vi "FTR Type DB Manager.vi"(5 "Command":T2, 6 "Local Data in":T3, 7 "UI Refs":T1, 8 "error in (no error)":errorcluster, 10 "Mouse Position (Start)":cluster{"X":i32, "Y":i32}) -> (0 "error out":errorcluster, 4 "Local Data out":T3)   [LabVIEW 2024]
uses:
  Controls/RVHR - Local Data.ctl
  Controls/Test Cluster.ctl
  Controls/Excluded Information.ctl
  Controls/Language.ctl
  Controls/Device_Type.ctl
  <vilib>/Utility/miscctls.llb/LVRectTypeDef.ctl
  <vilib>/Utility/miscctls.llb/LVBoundsTypeDef.ctl
  Controls/DB FTR Commands.ctl
  Controls/RVHR - UI Refs.ctl
  <vilib>/drjdpowell/SQLite Library/SQL Connection/Open (path).vi
  <vilib>/drjdpowell/SQLite Library/SQL Connection/Open (string).vi
  <vilib>/AdvancedString/Path To Command Line String.vi
  <vilib>/drjdpowell/SQLite Library/SQL Connection/Execute SQL.vi
  <vilib>/drjdpowell/SQLite Library/SQL Connection/Execute SQL (No results).vi
  <vilib>/drjdpowell/SQLite Library/SQL Connection/Execute SQL (Single Integer).vi
  <vilib>/drjdpowell/SQLite Library/SQL Connection/Connection.lvclass
  <vilib>/drjdpowell/SQLite Library/SQLite.lvlib
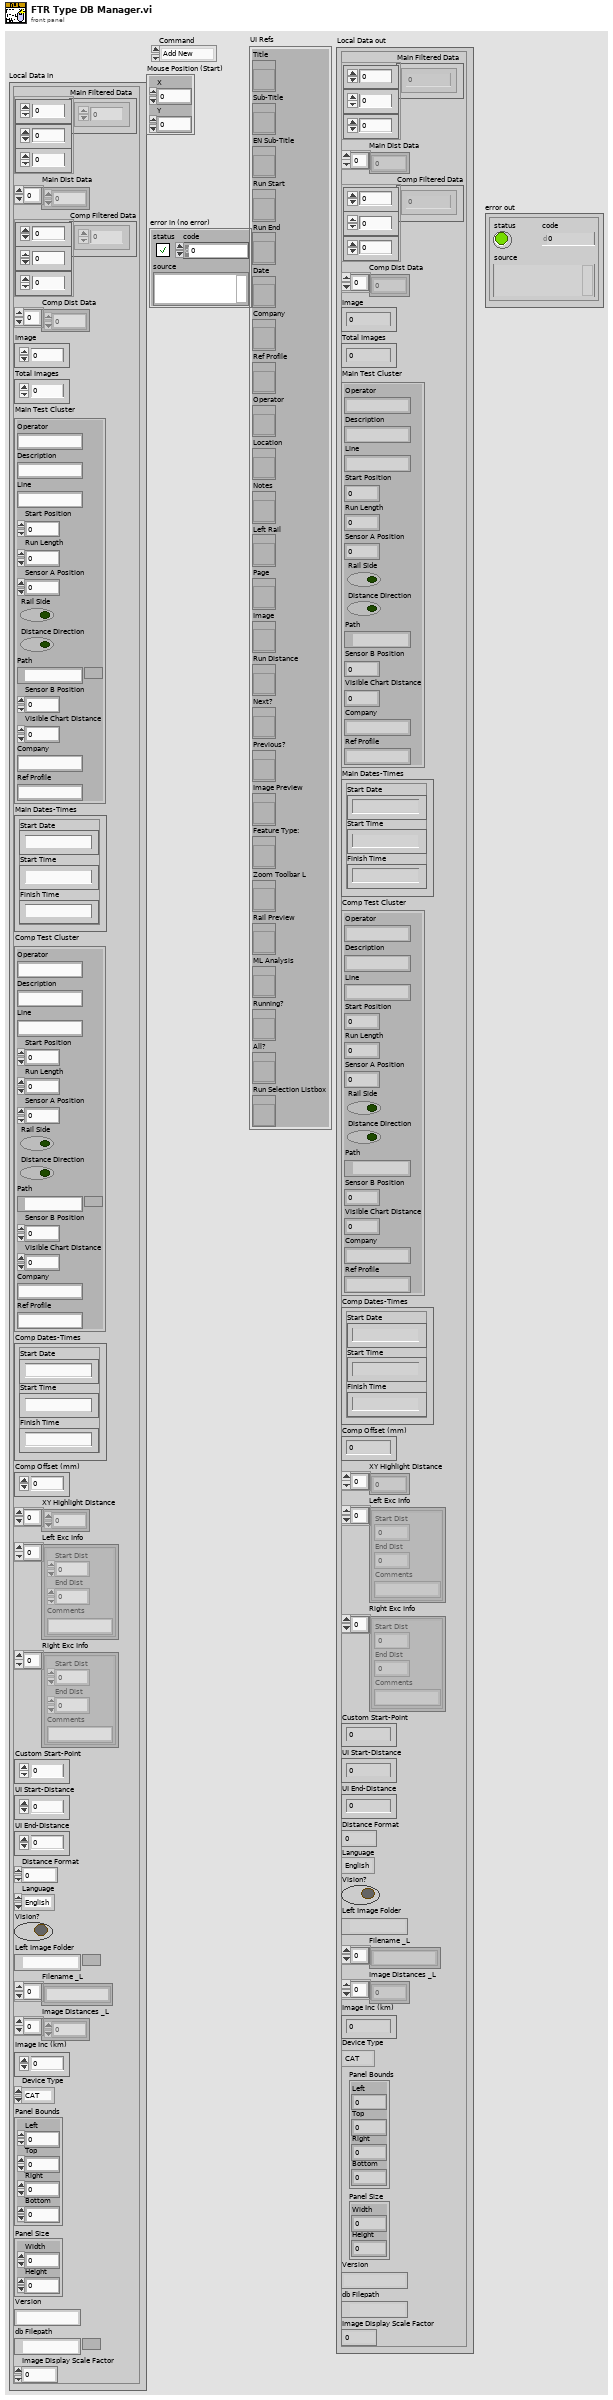
[diagram p1: front panel]
types:
  T1 = typedef "RVHR - UI Refs.ctl" = cluster{"Title":refnum<vi>, "Sub-Title":refnum<vi>, "EN Sub-Title":refnum<vi>, "Run Start":refnum<vi>, "Run End":refnum<vi>, "Date":refnum<vi>, "Company":refnum<vi>, "Ref Profile":refnum<vi>, "Operator":refnum<vi>, "Location":refnum<vi>, "Notes":refnum<vi>, "Left Rail":refnum<vi>, "Page":refnum<vi>, "Image":refnum<vi>, "Run Distance":refnum<vi>, "Next?":refnum<vi>, "Previous?":refnum<vi>, "Image Preview":refnum<vi>, "Feature Type:":refnum<vi>, "Zoom Toolbar L":refnum<vi>, "Rail Preview":refnum<vi>, "ML Analysis":refnum<vi>, "Running?":refnum<vi>, "All?":refnum<vi>, "Run Selection Listbox":refnum<vi>}
  T2 = typedef "DB FTR Commands.ctl" = enum16{"Add New", "Get", "Update"}
  T3 = typedef "RVHR - Local Data.ctl" = cluster{"Main Filtered Data":dbl[][][], "Main Dist Data":dbl[], "Comp Filtered Data":dbl[][][], "Comp Dist Data":dbl[], "Image":u16, "Total Images":u16, "Main Test Cluster":T4, "Main Dates-Times":cluster{"Start Date":string, "Start Time":string, "Finish Time":string}, "Comp Test Cluster":T4, "Comp Dates-Times":cluster{"Start Date":string, "Start Time":string, "Finish Time":string}, "Comp Offset (mm)":i64, "XY Highlight Distance":dbl[], "Left Exc Info":T5[], "Right Exc Info":T5[], "Custom Start-Point":dbl, "UI Start-Distance":dbl, "UI End-Distance":dbl, "Distance Format":u8, "Language":T6, "Vision?":bool, "Left Image Folder":path, "Filename _L":string[], "Image Distances _L":dbl[], "Image Inc (km)":dbl, "Device Type":T7, "Panel Bounds":T8, "Panel Size":T9, "Version":string, "db Filepath":path, "Image Display Scale Factor":dbl}
  T4 = typedef "Test Cluster.ctl" = cluster{"Operator":string, "Description":string, "Line":string, "Start Position":dbl, "Run Length":dbl, "Sensor A Position":dbl, "Rail Side":bool, "Distance Direction":bool, "Path":path, "Sensor B Position":dbl, "Visible Chart Distance":dbl, "Company":string, "Ref Profile":string}
  T5 = typedef "Excluded Information.ctl" = cluster{"Start Dist":dbl, "End Dist":dbl, "Comments":string}
  T6 = typedef "Language.ctl" = enum16{"English", "Chinese", "German"}
  T7 = typedef "Device_Type.ctl" = enum16{"CAT", "Bi-CAT", "YRCA", "RCA", "RV-HR", "TV-HR"}
  T8 = typedef "LVRectTypeDef.ctl" = cluster{"Left":i16, "Top":i16, "Right":i16, "Bottom":i16}
  T9 = typedef "LVBoundsTypeDef.ctl" = cluster{"Width":u32, "Height":u32}
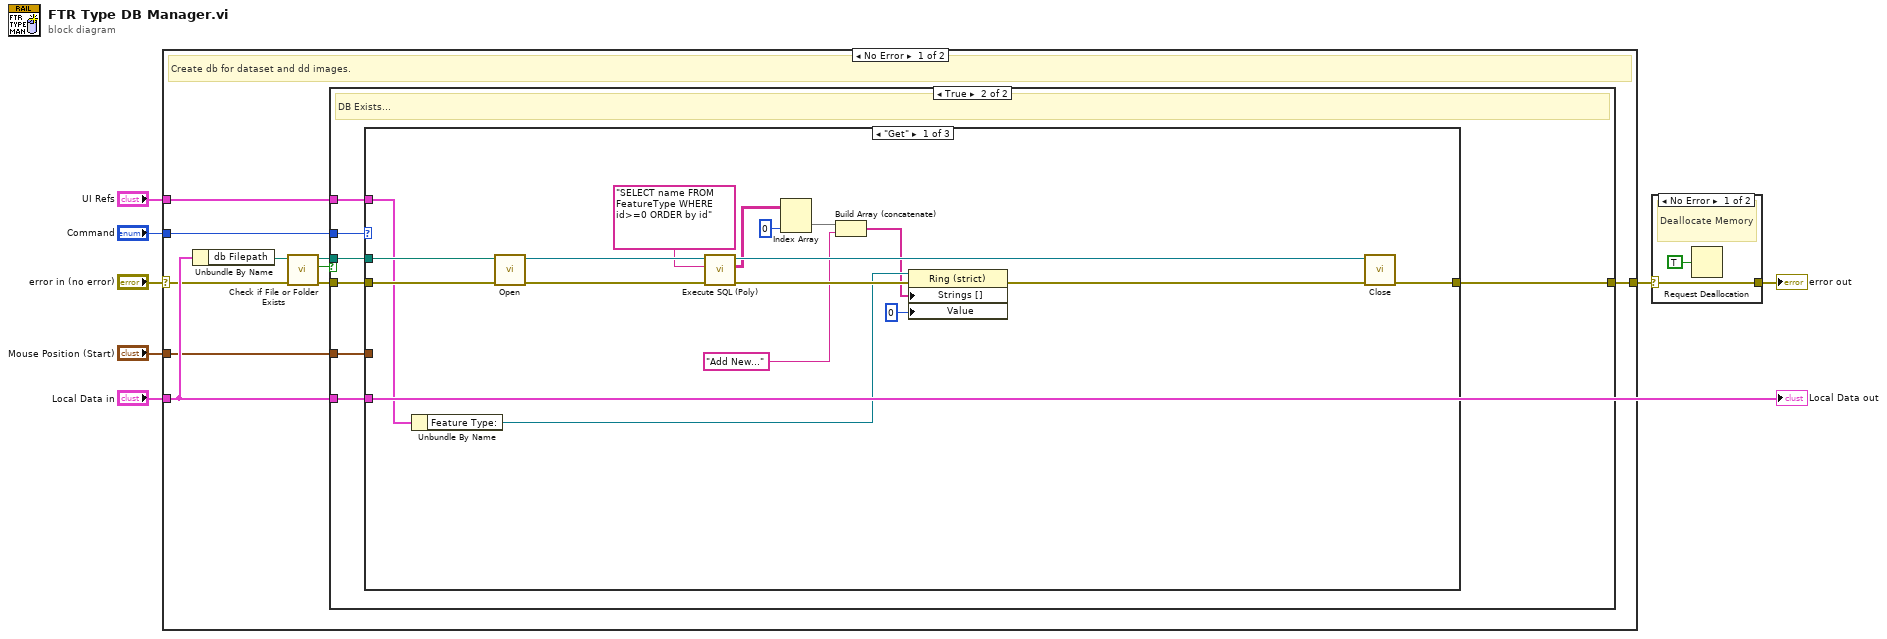
[diagram p0: block diagram]
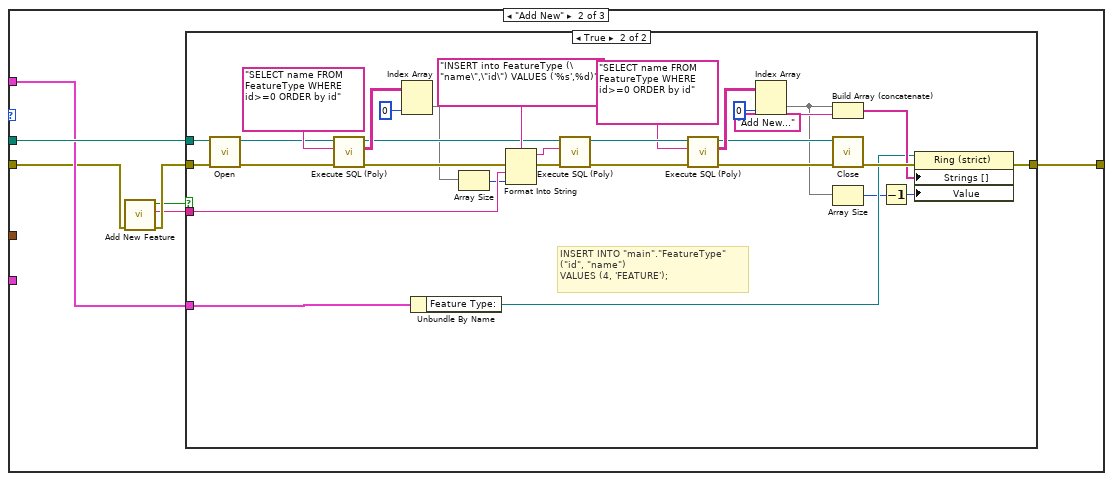
[diagram p4: hidden frame]
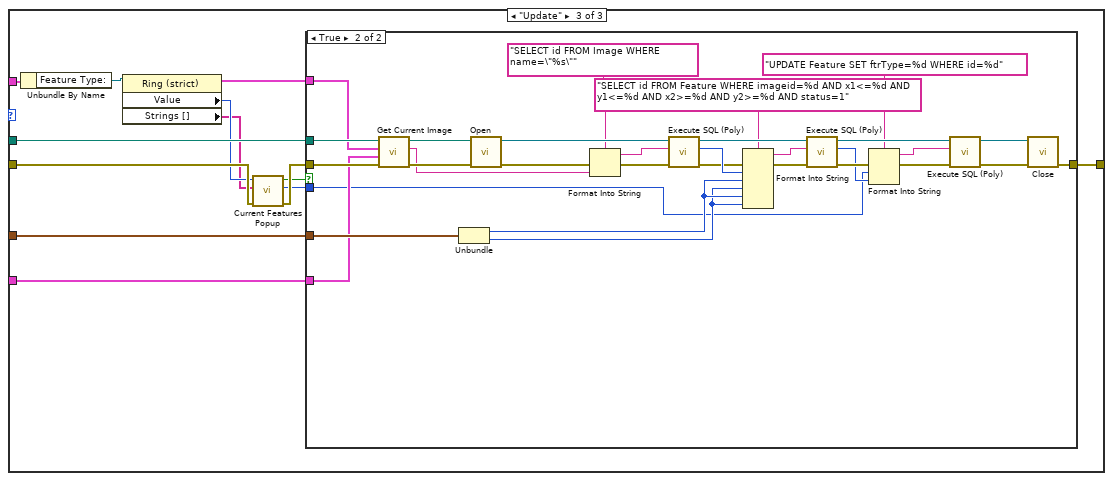
[diagram p6: hidden frame]
diagram:
  n1 = case shown="No Error" "error in (no error)" {
    selector: "error in (no error)" -> [w12 w124]
    tunnel: [w14 w124] -> w2
    tunnel: "Local Data in" -> [w13 _]
    tunnel: "Command" -> [w10 _]
    tunnel: "UI Refs" -> [w9 _]
    tunnel: "Mouse Position (Start)" -> [w8 _]
    frame No Error {
      # "Create db for dataset and dd images."
      n2 = Unbundle By Name(w13) -> ("db Filepath"=w11:path)
      n3 = call <vilib>:"Check if File or Folder Exists.vi"("error in (no error)"=w12, "path"=w11) -> ("error out"=w15:errorcluster, "file or folder exists?"=w17:bool, "dup path"=w16:path)  [unwired: 7 in]
      n4 = case shown="True" w17 {
        tunnel: w16 -> [_ w22]
        tunnel: w15 -> [w18 w23]
        tunnel: w13 -> [_ w25]
        tunnel: [w18 w24] -> w14
        tunnel: w10 -> [_ w21]
        tunnel: w9 -> [_ w20]
        tunnel: w8 -> [_ w19]
        frame False {
          # "Does not exist. Do nothing..."
        }
        frame True {
          # "DB Exists..."
          n5 = case shown="\"Get\"" w21 {
            tunnel: w25 -> [_ _ w81]
            tunnel: [w41 w49 w92] -> w24
            tunnel: w23 -> [w40 w46 w90]
            tunnel: w22 -> [w39 w48 w91]
            tunnel: w20 -> [w34 w47 w82]
            tunnel: w19 -> [_ _ w83]
            frame "Get" {
              n6 = Unbundle By Name(w34) -> ("Feature Type:"=w32:refnum<vi>)
              n7 = call-poly <vilib>:"Open.vi"("error in (no error)"=w40, "db file"=w39) -> ("error out"=w37:errorcluster, "SQLite Connection"=w42:refnum<class "Connection.lvclass">)  [unwired: 8 in]
              n8 = call-poly <vilib>:"Execute SQL (Poly).vi"("error in (no error)"=w37, "SQL"="SELECT name FROM FeatureType WHERE id>=0 ORDER by id" ("format string"), "SQLite Connection in"=w42) -> ("error out"=w35:errorcluster, "Result Set"=w30:string[][], "SQLite Connection"=w38:refnum<class "Connection.lvclass">)  [unwired: 5 in, 1 out]
              n9 = Index Array(array=w30, index (col)=0 ("disabled index (col)")) -> (element=w29:string[])  [unwired: 1 in]
              n10 = Build Array (concatenate)(w29, "Add New...") -> (w27:string[])
              n11 = property class="Ring (strict)"(reference=w32, error in=w35, "Strings []"=w27, "Value"=u16 0) -> (error out=w33:errorcluster)  [unwired: 1 out]
              n12 = call-dynamic "Close.vi"("error in (no error)"=w33, "SQLite Connection in"=w38) -> ("error out"=w41:errorcluster)  [unwired: 9 in]
            }
            frame "Add New" {
              n13 = call "Add New Feature.vi"("error in"=w46) -> ("error out"=w45:errorcluster, "New Feature"=w43:string, "Add New?"=w44:bool)  [unwired: 8 in]
              n14 = case shown="True" w44 {
                tunnel: [w50 w80] -> w49
                tunnel: w45 -> [w50 w79]
                tunnel: w48 -> [_ w78]
                tunnel: w47 -> [_ w69]
                tunnel: w43 -> [_ w67]
                frame False {
                }
                frame True {
                  # "INSERT INTO \"main\".\"FeatureType\"\n(\"id\", \"name\")\nVALUES (4, 'FEATURE');"
                  n15 = call-poly <vilib>:"Open.vi"("error in (no error)"=w79, "db file"=w78) -> ("error out"=w63:errorcluster, "SQLite Connection"=w64:refnum<class "Connection.lvclass">)  [unwired: 8 in]
                  n16 = call-poly <vilib>:"Execute SQL (Poly).vi"("error in (no error)"=w63, "SQL"="SELECT name FROM FeatureType WHERE id>=0 ORDER by id" ("format string"), "SQLite Connection in"=w64) -> ("error out"=w62:errorcluster, "Result Set"=w73:string[][], "SQLite Connection"=w61:refnum<class "Connection.lvclass">)  [unwired: 5 in, 1 out]
                  n17 = Index Array(array=w73, index (col)=0 ("disabled index (col)")) -> (element=w60:string[])  [unwired: 1 in]
                  n18 = Unbundle By Name(w69) -> ("Feature Type:"=w68:refnum<vi>)
                  n19 = Array Size(array=w60) -> (size(s)=w59:i32)
                  n20 = Format Into String(format string="INSERT into FeatureType (\"name\",\"id\") VALUES ('%s',%d)", error in=w62, w67, w59) -> (resulting string=w76:string, error out=w77:errorcluster)  [unwired: 1 in]
                  n21 = call-poly <vilib>:"Execute SQL (Poly).vi"("error in (no error)"=w77, "SQL"=w76, "SQLite Connection in"=w61) -> ("error out"=w54:errorcluster, "SQLite Connection"=w56:refnum<class "Connection.lvclass">)  [unwired: 7 in]
                  n22 = call-poly <vilib>:"Execute SQL (Poly).vi"("error in (no error)"=w54, "SQL"="SELECT name FROM FeatureType WHERE id>=0 ORDER by id" ("format string"), "SQLite Connection in"=w56) -> ("error out"=w53:errorcluster, "Result Set"=w57:string[][], "SQLite Connection"=w52:refnum<class "Connection.lvclass">)  [unwired: 5 in, 1 out]
                  n23 = Index Array(array=w57, index (col)=0 ("disabled index (col)")) -> (element=w51:string[])  [unwired: 1 in]
                  n24 = Build Array (concatenate)(w51, "Add New...") -> (w71:string[])
                  n25 = call-dynamic "Close.vi"("error in (no error)"=w53, "SQLite Connection in"=w52) -> ("error out"=w80:errorcluster)  [unwired: 9 in]
                  n26 = Array Size(array=w51) -> (size(s)=w66:i32)
                  n27 = Decrement(x=w66) -> (x-1=w65:i32)
                  n28 = property class="Ring (strict)"(reference=w68, "Strings []"=w71, "Value"=w65) -> ()  [unwired: 1 in, 2 out]
                }
              }
            }
            frame "Update" {
              n29 = Unbundle By Name(w82) -> ("Feature Type:"=w86:refnum<vi>)
              n30 = property class="Ring (strict)"(reference=w86) -> ("Value"=w85:u16, "Strings []"=w84:string[])  [unwired: 1 in, 2 out]
              n31 = call "Current Features Popup.vi"("error in"=w90, "Strings []"=w84, "Feature Type:"=w85) -> ("error out"=w89:errorcluster, "Feature Type: 2"=w87:u16, "Update?"=w88:bool)  [unwired: 6 in]
              n32 = case shown="True" w88 {
                tunnel: [w93 w101] -> w92
                tunnel: w89 -> [w93 w100]
                tunnel: w91 -> [_ w99]
                tunnel: w87 -> [_ w94]
                tunnel: w83 -> [_ w98]
                tunnel: w82 -> [_ w97]
                tunnel: w81 -> [_ w96]
                frame False {
                }
                frame True {
                  n33 = call "Get Current Image.vi"("error in (no error)"=w100, "Local Data in"=w96, "UI References"=w97) -> ("error out"=w123:errorcluster, "Current Image"=w110:string)  [unwired: 7 in]
                  n34 = Unbundle(w98) -> ("X"=w115:i32, "Y"=w114:i32)
                  n35 = call-poly <vilib>:"Open.vi"("error in (no error)"=w123, "db file"=w99) -> ("error out"=w113:errorcluster, "SQLite Connection"=w108:refnum<class "Connection.lvclass">)  [unwired: 8 in]
                  n36 = Format Into String(format string="SELECT id FROM Image WHERE name=\"%s\"", error in=w113, w110) -> (resulting string=w107:string, error out=w111:errorcluster)  [unwired: 1 in]
                  n37 = call-poly <vilib>:"Execute SQL (Poly).vi"("error in (no error)"=w111, "SQL"=w107, "SQLite Connection in"=w108) -> ("error out"=w112:errorcluster, "Result"=w121:i64, "SQLite Connection"=w109:refnum<class "Connection.lvclass">)  [unwired: 6 in]
                  n38 = Format Into String(format string="SELECT id FROM Feature WHERE imageid=%d AND x1<=%d AND y1<=%d AND x2>=%d AND y2>=%d AND status=1", error in=w112, w121, w115, w114, w115, w114) -> (resulting string=w106:string, error out=w105:errorcluster)  [unwired: 1 in]
                  n39 = call-poly <vilib>:"Execute SQL (Poly).vi"("error in (no error)"=w105, "SQL"=w106, "SQLite Connection in"=w109) -> ("error out"=w118:errorcluster, "Result"=w95:i64, "SQLite Connection"=w116:refnum<class "Connection.lvclass">)  [unwired: 6 in]
                  n40 = Format Into String(format string="UPDATE Feature SET ftrType=%d WHERE id=%d", error in=w118, w94, w95) -> (resulting string=w122:string, error out=w119:errorcluster)  [unwired: 1 in]
                  n41 = call-poly <vilib>:"Execute SQL (Poly).vi"("error in (no error)"=w119, "SQL"=w122, "SQLite Connection in"=w116) -> ("error out"=w120:errorcluster, "SQLite Connection"=w117:refnum<class "Connection.lvclass">)  [unwired: 7 in]
                  n42 = call-dynamic "Close.vi"("error in (no error)"=w120, "SQLite Connection in"=w117) -> ("error out"=w101:errorcluster)  [unwired: 9 in]
                }
              }
            }
          }
        }
      }
    }
    frame Error {
    }
  }
  n43 = case shown="No Error" w2 {
    selector: w2 -> [w125 w127]
    tunnel: [w125 w127] -> w1
    frame No Error {
      # "Deallocate Memory"
      n44 = Request Deallocation(TRUE ("flag")) -> ()
    }
    frame Error {
    }
  }
  "error out" <- w1
  "Local Data out" <- "Local Data in"
